vi "Charger_Multi-Channel Init Panel.vi"(5 "Status Refnum  Array":T1[](array[typedef]), 6 "error in":errorcluster) -> (0 "error out":errorcluster)   [LabVIEW 2020]
doc: "This function initializes the Charger Multi-Chanel panel attributes including default values and control colors."
uses:
  Charger_Status Refnum.ctl
  Drivers/Charger Test Set/Charger_Input Control.ctl
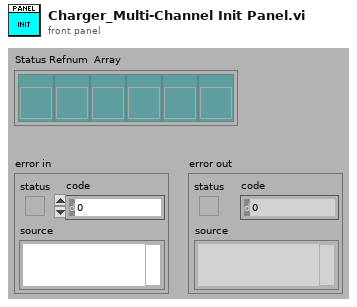
[diagram p1: front panel]
types:
  T1 = typedef "Charger_Status Refnum.ctl" = refnum<vi>
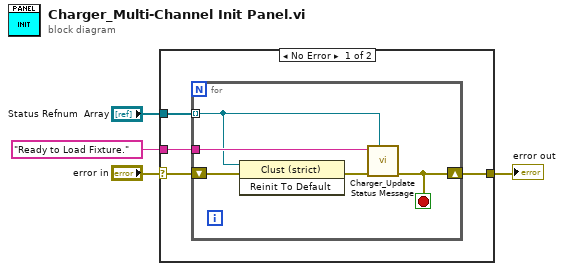
[diagram p0: block diagram]
diagram:
  n1 = case shown="No Error" "error in" {
    selector: "error in" -> [w8 w14]
    tunnel: [w5 w14] -> w4
    tunnel: "Status Refnum  Array" -> [w6 _]
    tunnel: "Ready to Load Fixture." -> [w7 _]
    frame No Error {
      n2 = for {
        shift-right: [w12] -> w5
        shift-left: w8 -> [w11]
        tunnel: w7 -> [w13]
        tunnel: w6 -> [w9] mode=indexing
        stop <- w12 stop-if-true
        n3 = invoke class="Clust (strict)" method="Reinit To Default"(reference=w9, error in=w11) -> (error out=w10:errorcluster)  [unwired: 1 in, 2 out]
        n4 = call "Charger_Update Status Message.vi"("Status Refnum"=w9, "error in"=w10, "status message"=w13) -> ("error out"=w12:errorcluster)  [unwired: 6 in]
      }
    }
    frame Error {
    }
  }
  "error out" <- w4
